vi "FPGA Main Sine Test.vi"   [LabVIEW 2018]
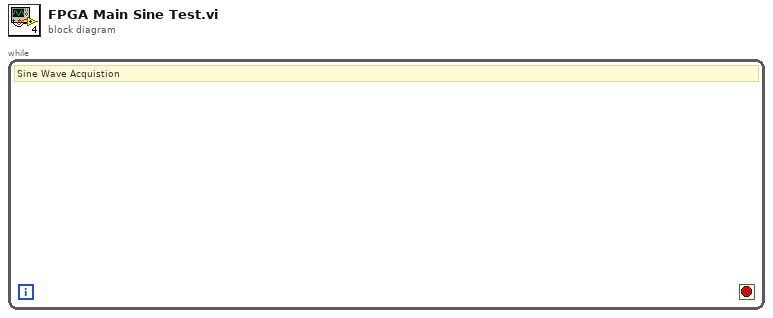
[diagram p0: block diagram]
diagram:
  n1 = while {
    stop <- _ stop-if-true
    # "Sine Wave Acquistion"
  }
